vi "Configure Write Command Msg Timeout.vi"(10 "Message Timeout in":i32) -> (2 "Message Timeout out":i32)   [LabVIEW 2017, in "SSH.lvlib"]
doc: "Allows the user to set a timeout longer than the default 5 seconds if needed."
uses:
  SSH.lvlib
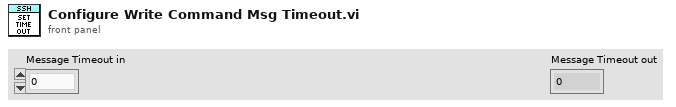
[diagram p1: front panel]
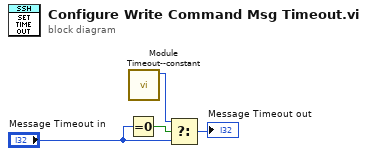
[diagram p0: block diagram]
diagram:
  n1 = Equal To 0?(x="Message Timeout in") -> (x = 0?=w4:bool)
  n2 = call "Module Timeout--constant.vi"() -> ("Module Timeout"=w3:i32)  [unwired: 11 in]
  n3 = Select(t=w3, s=w4, f="Message Timeout in") -> (s? t:f=→"Message Timeout out":i32)
